vi "HostDynamicRetractFormalization.vi"(6 "Retract_Edge um":dbl format="%#_13g", 7 "Retract_Flat um":dbl format="%#_13g", 8 "YNum":i32, 9 "XNum":i32, 11 "InputLabel":dbl[][](array[numeric])) -> (3 "OutputRetractMap um":dbl[][](array[numeric]))   [LabVIEW 2024]
uses:
  <vilib>/gmath/interp.llb/Interpolate 2D (1d xi,yi).vi
  <vilib>/gmath/NI_Gmath.lvlib
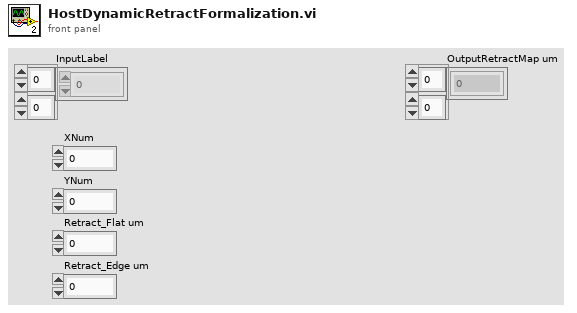
[diagram p1: front panel]
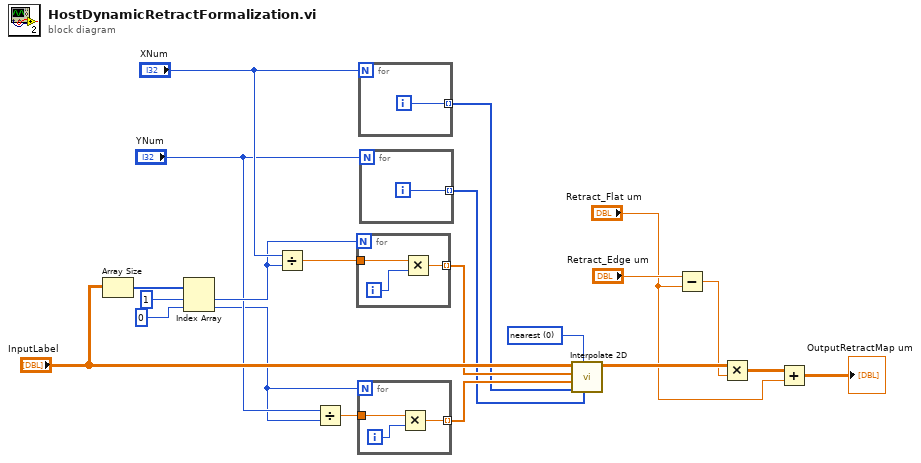
[diagram p0: block diagram]
diagram:
  w20 = 0 items=["nearest", "bilinear", "bicubic", "bicubic spline"] ("method")
  n1 = Array Size(array="InputLabel") -> (size(s)=w17:i32[])
  n2 = Index Array(array=w17, index #1=1 ("index"), index #2=0 ("index")) -> (element #1=w13:i32, element #2=w11:i32)
  n3 = Divide(x="XNum", y=w13) -> (x/y=w14:dbl)
  n4 = Divide(x="YNum", y=w11) -> (x/y=w10:dbl)
  n5 = for {
    N: w13 -> [_]
    tunnel: w14 -> [w24]
    tunnel: [w22] -> w9 mode=indexing
    i -> [w23]
    n6 = Multiply(x=w24, y=w23) -> (x*y=w22:dbl)
  }
  n7 = for {
    N: w11 -> [_]
    tunnel: w10 -> [w27]
    tunnel: [w25] -> w8 mode=indexing
    i -> [w26]
    n8 = Multiply(x=w27, y=w26) -> (x*y=w25:dbl)
  }
  n9 = for {
    N: "XNum" -> [_]
    tunnel: [w28] -> w7 mode=indexing
    i -> [w28]
  }
  n10 = for {
    N: "YNum" -> [_]
    tunnel: [w29] -> w6 mode=indexing
    i -> [w29]
  }
  n11 = call-poly <vilib>:"Interpolate 2D.vi"("yi"=w6, "method"=w20, "xi"=w7, "Y"=w8, "X"=w9, "Z"="InputLabel") -> ("zi"=w5:dbl[][])  [unwired: 2 in, 3 out]
  n12 = Subtract(x="Retract_Edge um", y="Retract_Flat um") -> (x-y=w4:dbl)
  n13 = Multiply(x=w5, y=w4) -> (x*y=w3:dbl[][])
  n14 = Add(x=w3, y="Retract_Flat um") -> (x+y=→"OutputRetractMap um":dbl[][])
